vi "DB Select data(Count index).vi"(6 "index":i32, 7 "Condtion":string, 8 "error in (no error)":errorcluster caption="错误输入（无错误）", 9 "Code":string, 10 "Tabe":string, 11 "Connncet State":T1) -> (0 "error out":errorcluster caption="错误输出", 1 "Count":i32, 2 "state":bool, 3 "Connncet State out":T1)   [LabVIEW 2014]
uses:
  <vilib>/addons/database/NI_Database_API.lvlib
  Ctr/Constr.ctl
  <vilib>/addons/database/Connection.llb/Conn ObjectReference.ctl
  Ctr/Conneect State.ctl
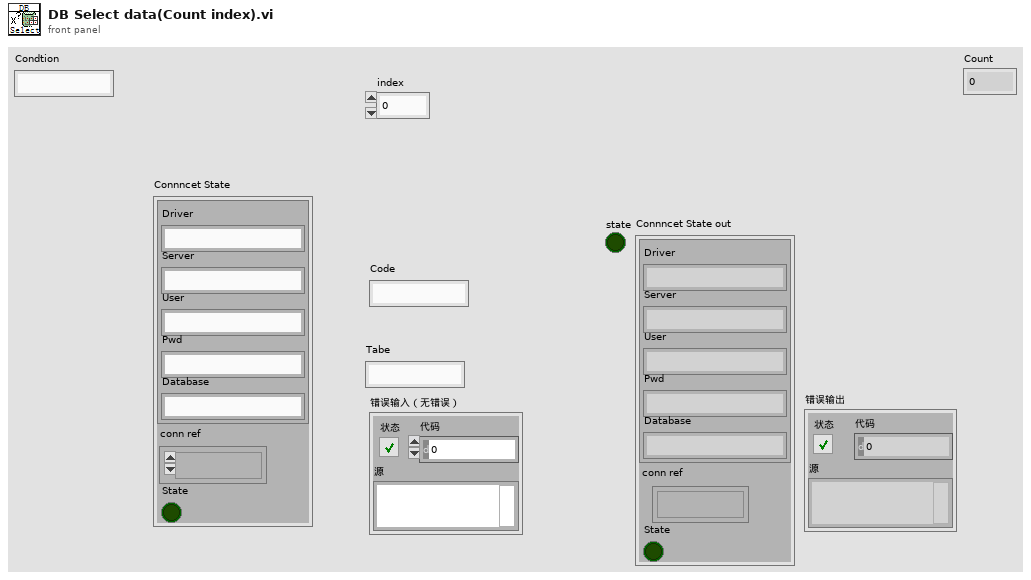
[diagram p1: front panel]
types:
  T1 = typedef "Conneect State.ctl" = cluster{"Constr":T2, "conn ref":T3, "State":bool}
  T2 = typedef "Constr.ctl" = cluster{"Driver":string, "Server":string, "User":string, "Pwd":string, "Database":string}
  T3 = typedef "NI_Database_API.lvlib/Conn ObjectReference.ctl" = refnum<k1>
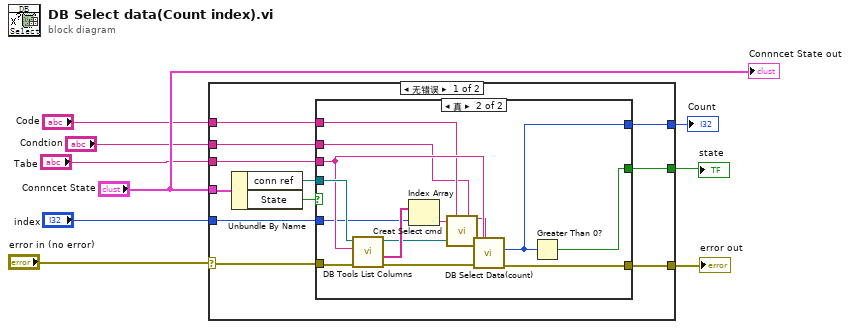
[diagram p0: block diagram]
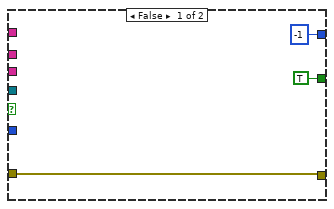
[diagram p2: hidden frame]
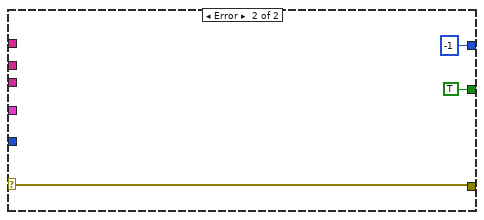
[diagram p3: hidden frame]
diagram:
  n1 = case shown="无错误" "error in (no error)" {
    selector: "error in (no error)" -> [w18 w40]
    tunnel: "Connncet State" -> [w20 _]
    tunnel: "Tabe" -> [w16 _]
    tunnel: "Code" -> [w15 _]
    tunnel: [w14 w40] -> w5
    tunnel: [w13 TRUE] -> w4
    tunnel: "index" -> [w12 _]
    tunnel: [w11 -1 ("Count")] -> w2
    tunnel: "Condtion" -> [w10 _]
    frame No Error {
      n2 = Unbundle By Name(w20) -> ("conn ref"=w17:T3, "State"=w19:bool)
      n3 = case shown="真" w19 {
        tunnel: w18 -> [w23 w36]
        tunnel: w17 -> [_ w35]
        tunnel: w16 -> [_ w34]
        tunnel: w15 -> [_ w32]
        tunnel: [w23 w37] -> w14
        tunnel: [TRUE w26] -> w13
        tunnel: w12 -> [_ w27]
        tunnel: [-1 ("Count") w25] -> w11
        tunnel: w10 -> [_ w24]
        frame False {
        }
        frame True {
          n4 = call <vilib>:"DB Tools List Columns.vi"("error in (no error)"=w36, "table"=w34, "connection reference"=w35) -> ("error out"=w33:errorcluster, "columns"=w30:string[], "connection reference out"=w29:T3)  [unwired: 1 in, 1 out]
          n5 = Index Array(array=w30, index=w27) -> (element=w28:string)
          n6 = call "Creat Select cmd.vi"("Col"=w28, "Code"=w32, "Condtion"=w24) -> ("Str"=w31:string)  [unwired: 11 in, 1 out]
          n7 = call "DB Select Data(count).vi"("condition"=w31, "error in (no error)"=w33, "table"=w34, "connection reference"=w29) -> ("error out"=w37:errorcluster, "Count"=w25:i32)  [unwired: 5 in, 1 out]
          n8 = Greater Than 0?(x=w25) -> (x > 0?=w26:bool)
        }
      }
    }
    frame Error {
    }
  }
  "error out" <- w5
  "state" <- w4
  "Count" <- w2
  "Connncet State out" <- "Connncet State"
